vi "intake-shooter.vi"() -> ()   [LabVIEW 2023]
uses:
  ctrl defs/ctrl shooter speeds.ctl
  ctrl defs/ctrl intake speeds.ctl
  ctrl defs/ctrl INTAKE STATES.ctl
  ctrl defs/ctrl SHOOTER STATES.ctl
  <vilib>/Rock Robotics/WPI/MotorControl/WPI_MotorControlDeviceRef.ctl
  <vilib>/Rock Robotics/WPI/MotorControl/WPI_MotorControlType.ctl
  <vilib>/Rock Robotics/SystemInterfaces/DIO/FPGA_DIOPWMChannel.ctl
  <vilib>/Rock Robotics/WPI/PWM/WPI_PWMDeadband.ctl
  <vilib>/Rock Robotics/SystemInterfaces/DIO/FPGA_DIOChannel.ctl
  <vilib>/Rock Robotics/WPI/ThirdParty/REV Robotics/REVLib/Typedef/Spark MAX Control Type.ctl
  Global INIT.vi
  Global stack names.vi
  <vilib>/Rock Robotics/Network Tables/NT Write String.vi
  <vilib>/Rock Robotics/Network Tables/NT Read Boolean.vi
  <vilib>/Rock Robotics/Network Tables/NT Write Boolean.vi
panel:
  in  "AUTO run\nINTAKE after\nSHOT":bool
  in  "WRITE to global":bool
  in  "reload global values":bool
  in  "LOADER speeds":T1={"forward"=0.64, "reverse"=-1.0} {"reverse" min=-1.0 max=-0.02 format="%.3f"; "forward" min=0.02 max=1.0 format="%.3f"}
  in  "LOADER max/min":T1={"forward"=0.75, "reverse"=-0.75} {"reverse" min=-1.0 max=-0.02 format="%.3f"; "forward" min=0.02 max=1.0 format="%.3f"}
  in  "INTAKE speeds":T1={"forward"=1.0, "reverse"=-0.75} {"reverse" min=-1.0 max=-0.02 format="%.3f"; "forward" min=0.02 max=1.0 format="%.3f"}
  in  "SHOOTER speeds":T2={"SPEAKER"=1.0, "AMP"=0.5} {"AMP" min=0.02 max=1.0 format="%.3f"; "SPEAKER" min=0.02 max=1.0 format="%.3f"}
  in  "milliseconds to wait\nREV LOADER":u32=125
  in  "wait for SHOOT\nto end (ms)":u32=500
  in  "wait to\nSPIN UP\nSHOOTER (ms)":u32=250
  in  "OVERIDE\nNOTE check for\nSHOOT":bool
  out "LOOKING\nfor NOTE":bool
  out "note sensor":bool
  in  "SHOOT STATUS":string="STANDBY"
  out "% TARGET\nSPEED":dbl=-0.0
  out "Set SHOOTER\nRPM":dbl=1419.0 format="%#_13g"
  out "max rpm\n- SHOOTER":dbl=1419.0
  out "FIRE!":bool
  in  "INTAKE STATUS":string="Standby"
  out "max rpm\n- INTAKE":dbl=1419.0
  out "NOTE is\nloaded":bool
  out "run reverse":bool
  out "run intake":bool
  out "run? is\nACTIVE":bool
  in  "milliseconds to wait\nIN REVERSE":u32=1000
  in  "milliseconds to wait\nafter NOTE trigger":u32=25
  out "EXT FLAP":bool
  out "AMP OPT":bool
  in  "REVS to\nSHOOT":dbl=5.0 format="%#_13g"
  in  "REVS to\nRETRACT":dbl=-1.0 format="%#_13g"
  out "max rpm\n- LOADER":dbl=1419.0
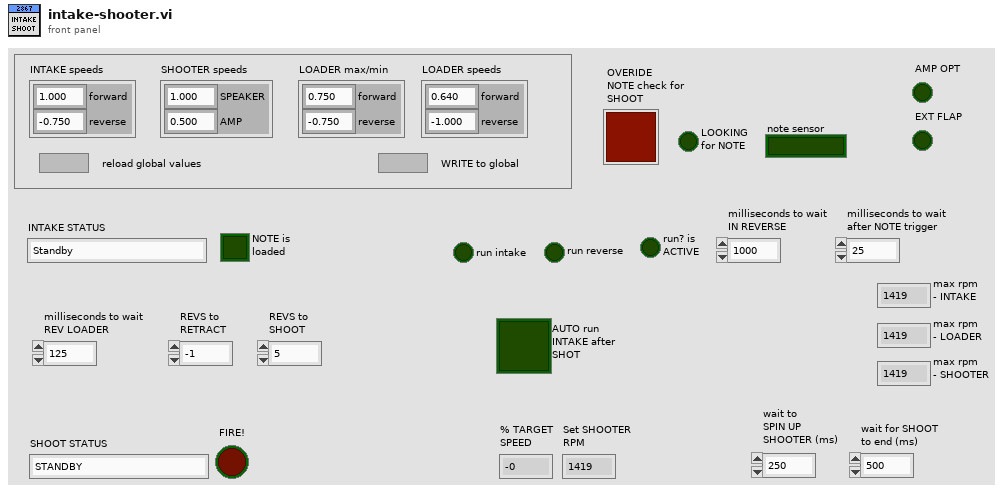
[diagram p1: front panel]
types:
  T1 = typedef "ctrl intake speeds.ctl" = cluster{"forward":dbl, "reverse":dbl}
  T2 = typedef "ctrl shooter speeds.ctl" = cluster{"SPEAKER":dbl, "AMP":dbl}
  T3 = typedef "ctrl SHOOTER STATES.ctl" = enum16{"STANDBY", "RETRACT NOTE", "SPIN-UP", "SHOOT", "RESET"}
  T4 = typedef "ctrl INTAKE STATES.ctl" = enum16{"STANDBY", "START INTAKES", "WATCH for NOTE", "SHUT DOWN", "REVERSE"}
  T5 = typedef "WPI_MotorControlDeviceRef.ctl" = cluster{"DeviceStatus":errorcluster, "Type":T6, "PWM":cluster{"PWM Channel":T7, "DeadBand":T8}, "CAN":cluster{"Device Number":u8, "SetOutput VI Ref":variant, "GetOutput VI Ref":variant, "Enable VI Ref":variant, "Disable VI Ref":variant, "Data":variant}, "Invert":bool, "DIO PWM":cluster{"PWM \"Enable\" Channel":T7, "DIOChannel":T9, "PWM Rate":dbl}}
  T6 = typedef "WPI_MotorControlType.ctl" = enum16{"PWM", "CAN", "DIO PWM"}
  T7 = typedef "FPGA_DIOPWMChannel.ctl" = enum8{"PWM 0", "PWM 1", "PWM 2", "PWM 3", "PWM 4", "PWM 5", "PWM 6", "PWM 7", "PWM 8", "PWM 9", "PWM MXP 0", "PWM MXP 1", "PWM MXP 2", "PWM MXP 3", "PWM MXP 4", "PWM MXP 5", "PWM MXP 6", "PWM MXP 7", "PWM MXP 8", "PWM MXP 9", "Invalid"}
  T8 = typedef "WPI_PWMDeadband.ctl" = cluster{"Name":string, "maxPositivePwm":i32, "minPositivePwm":i32, "centerPwm":i32, "maxNegativePwm":i32, "minNegativePwm":i32, "angularRange":u16}
  T9 = typedef "FPGA_DIOChannel.ctl" = enum8{"DIO 0", "DIO 1", "DIO 2", "DIO 3", "DIO 4", "DIO 5", "DIO 6", "DIO 7", "DIO 8", "DIO 9", "DIO MXP 0", "DIO MXP 1", "DIO MXP 2", "DIO MXP 3", "DIO MXP 4", "DIO MXP 5", "DIO MXP 6", "DIO MXP 7", "DIO MXP 8", "DIO MXP 9", "DIO MXP 10", "DIO MXP 11", "DIO MXP 12", "DIO MXP 13", "DIO MXP 14", "DIO MXP 15", "SPI Port CS1", "SPI Port CS2", "SPI Port CS3", "SPI Port MISO", "SPI Port MOSI", "Invalid"}
  T10 = cluster{"INTAKE ref":T5, "LOADER ref":T5, "SHOOTER ref":T5}
  T11 = typedef "ctrl DIO.ctl" = cluster{"description":string, "Installed?":bool, "DIOChannel":T9, "refnum name":string}
  T12 = typedef "ctrl swerve motor.ctl" = cluster{"description":string, "MOTOR SELECT":T13, "Installed?":bool, "CAN ID":u8, "refnum name":string, "Invert":bool, "Idle Mode":T14, "Current limiting":T15, "MOTOR PIDF coefficients":T16, "gear ratio":dbl}
  T13 = typedef "ctrl MOTOR SELECT.ctl" = i16
  T14 = typedef "Spark MAX Idle Mode.ctl" = enum16{"Coast", "Brake"}
  T15 = typedef "ctrl Spark MAX current limiting.ctl" = cluster{"Linearized":bool, "Free Speed (A)":dbl, "Primay (A)":dbl, "Limit RPM (0)":u32}
  T16 = typedef "ctrl motor PIDF coefficients.ctl" = cluster{"PIDF":cluster{"P Gain":dbl, "I Gain":dbl, "D Gain":dbl, "F Gain":dbl, "I Zone":dbl, "Min Output":dbl, "Max Output":dbl}, "Smart Motion":T17}
  T17 = typedef "Spark MAX Smart Motion Parameters.ctl" = cluster{"Max Velocity":dbl, "Max Acceleration":dbl, "Minimum Velocity Output":dbl, "Allowed Closed Loop Error":dbl}
  T18 = typedef "WPI_DigitalInputDevRef.ctl" = cluster{"DevStatus":errorcluster, "DIO Channel":T9}
  T19 = typedef "ctrl stack - INTAKE SHOOTER.ctl" = cluster{"INTAKE STATE":string, "RUN INTAKE?":string, "RUN REVERSE?":string, "NOTE LOADED?":string, "SHOOTER STATE":string, "SHOOTER FIRE?":string, "SHOOT AMP?":string, "EXTEND FLAP?":string, "LOOKING for NOTE":string}
  T20 = typedef "Spark MAX Control Type.ctl" = enum16{"Percent VBus", "Voltage", "Velocity", "Position", "Smart Motion", "Current", "Smart Velocity"}
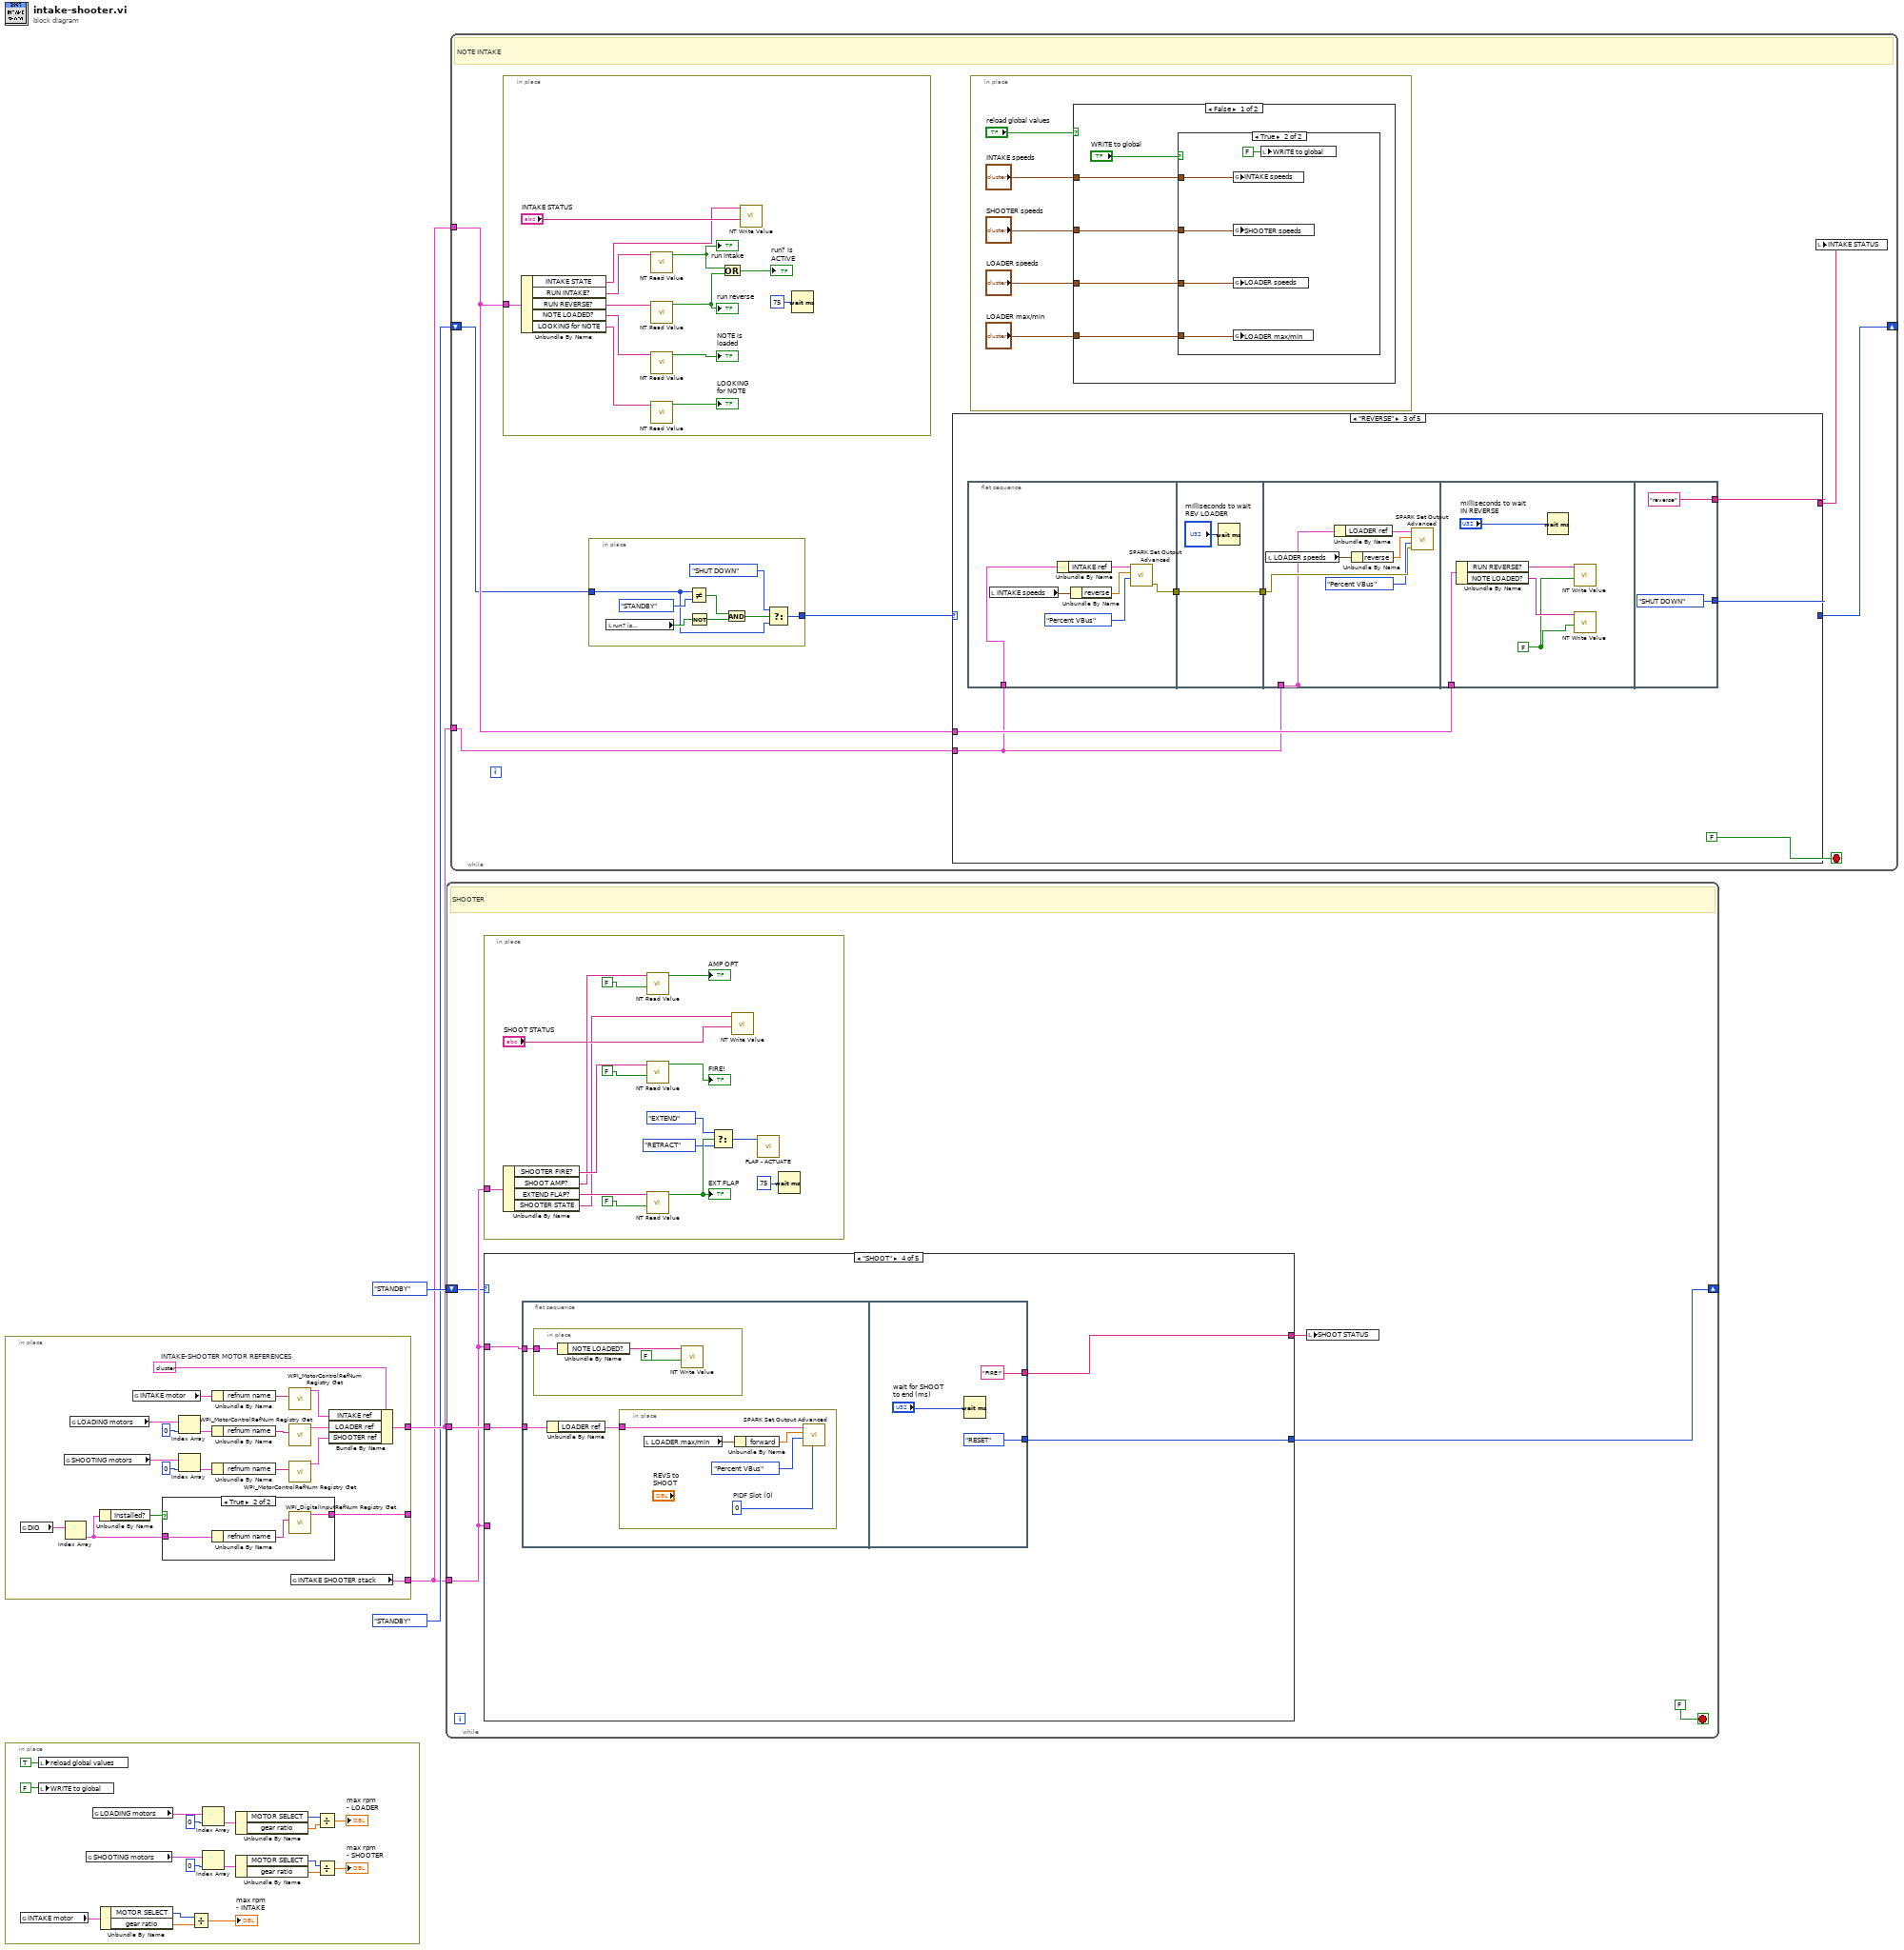
[diagram p0: block diagram]
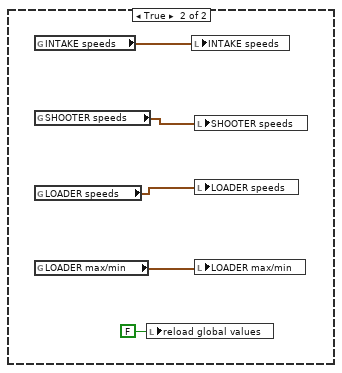
[diagram p3: hidden frame]
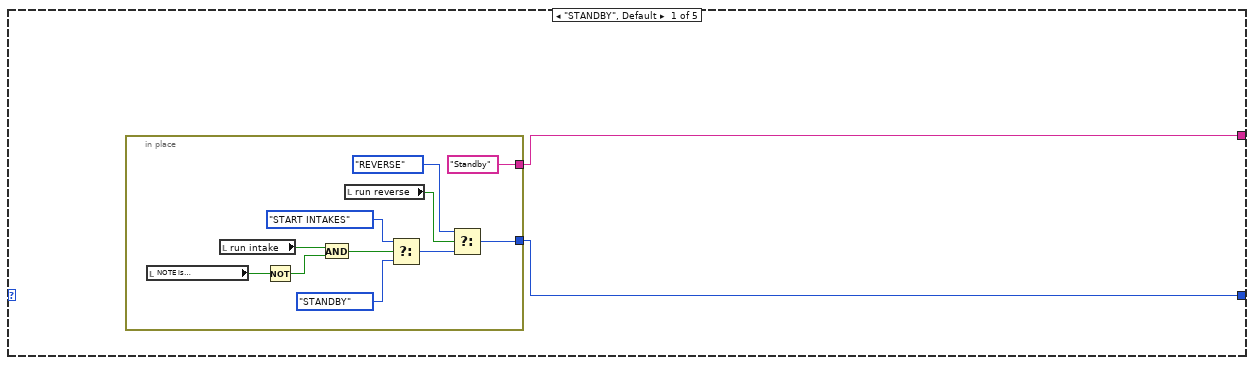
[diagram p4: hidden frame]
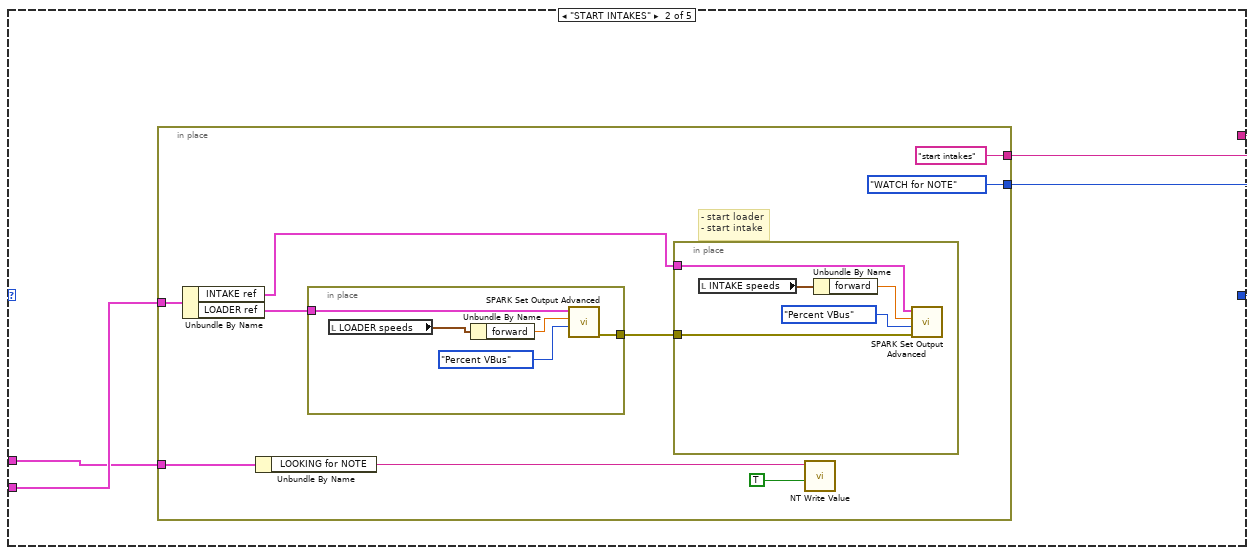
[diagram p5: hidden frame]
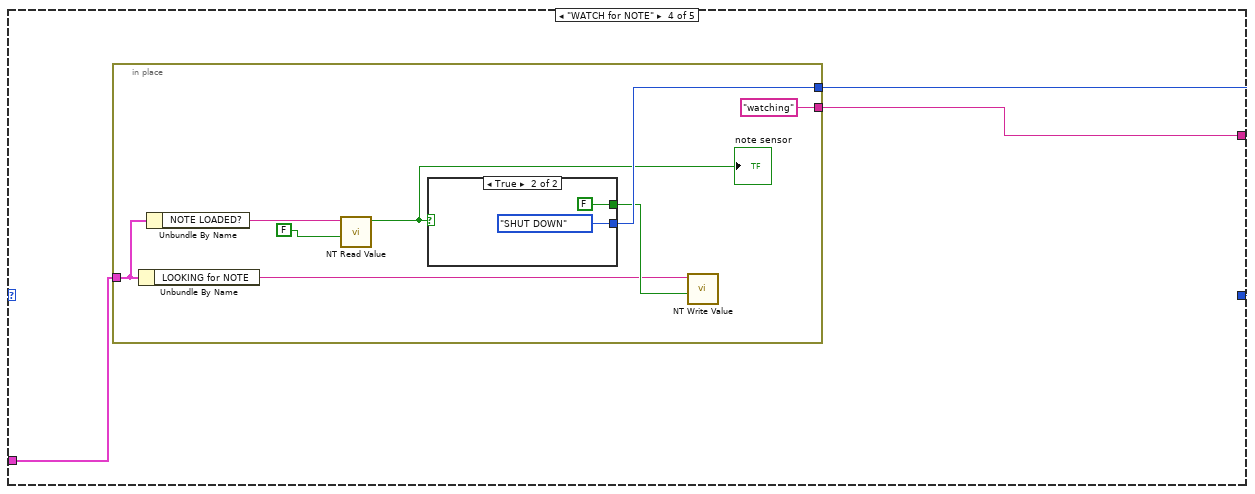
[diagram p6: hidden frame]
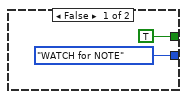
[diagram p7: hidden frame]
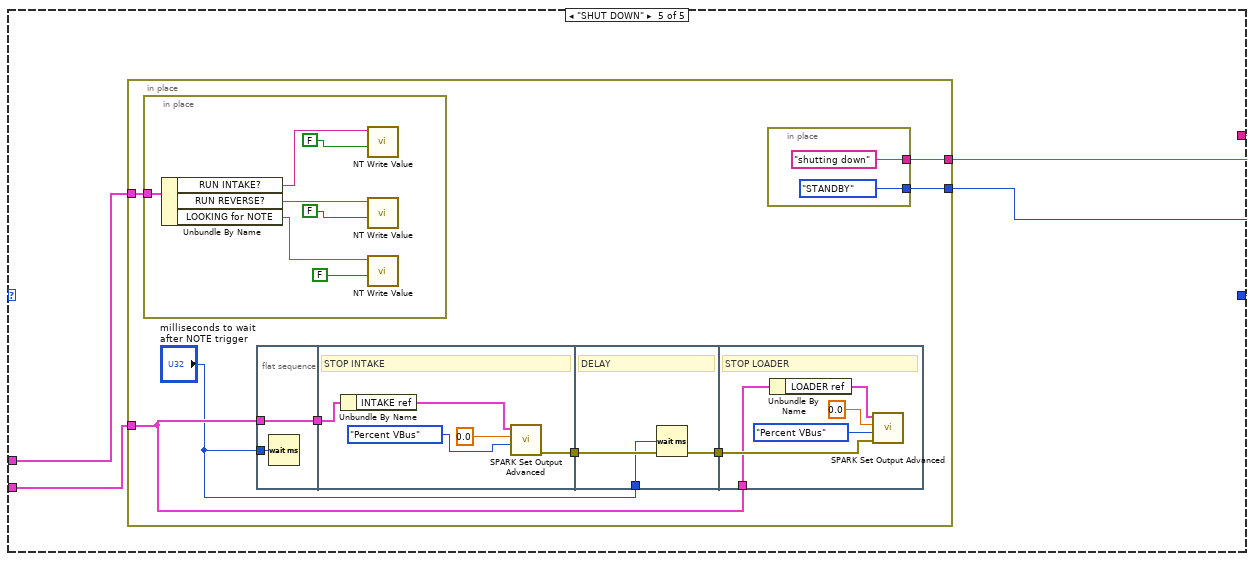
[diagram p8: hidden frame]
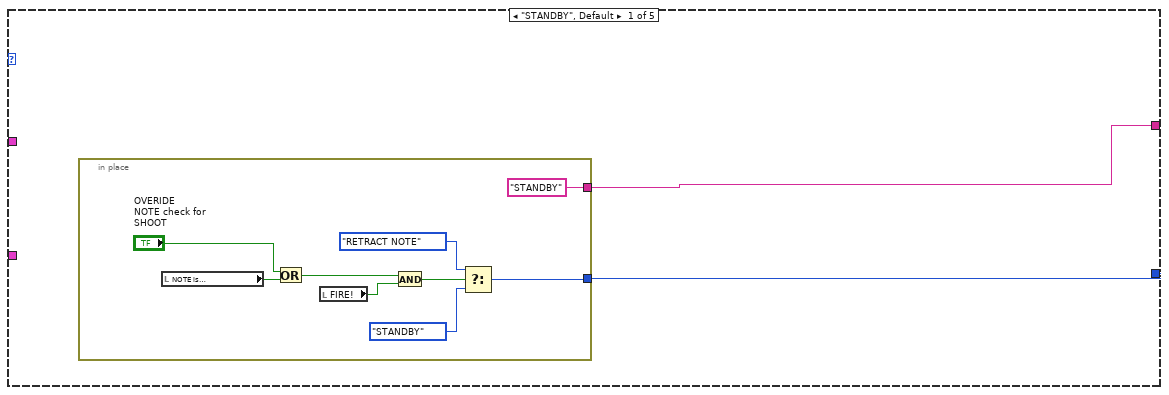
[diagram p9: hidden frame]
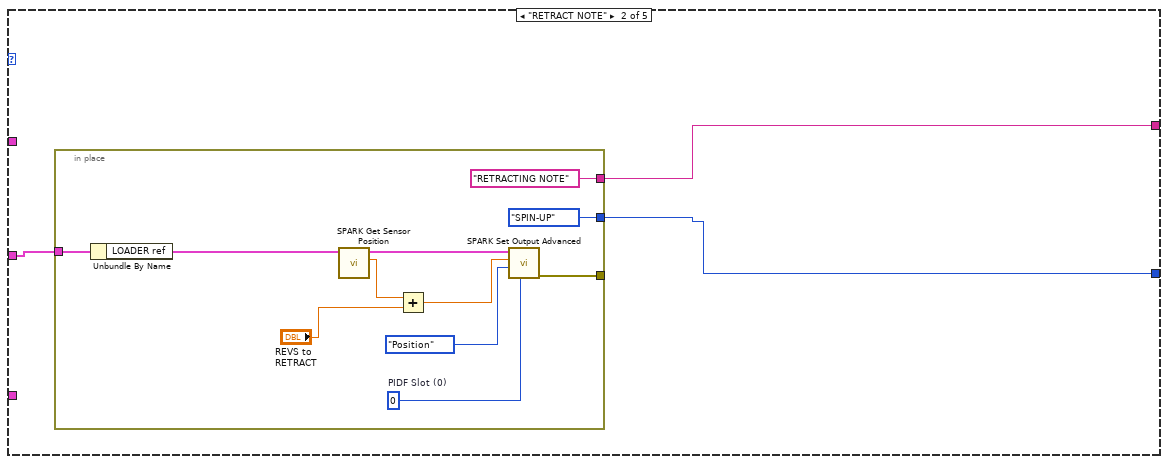
[diagram p10: hidden frame]
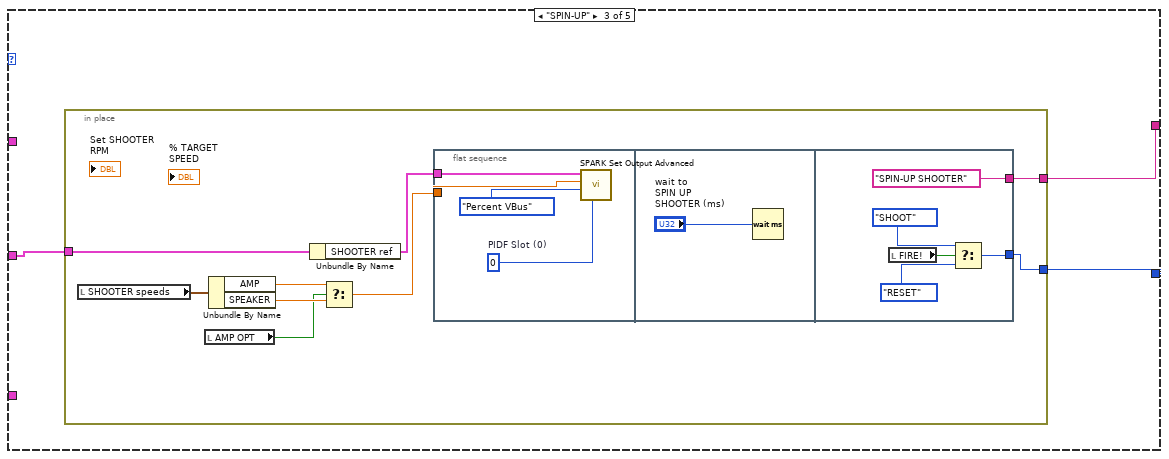
[diagram p11: hidden frame]
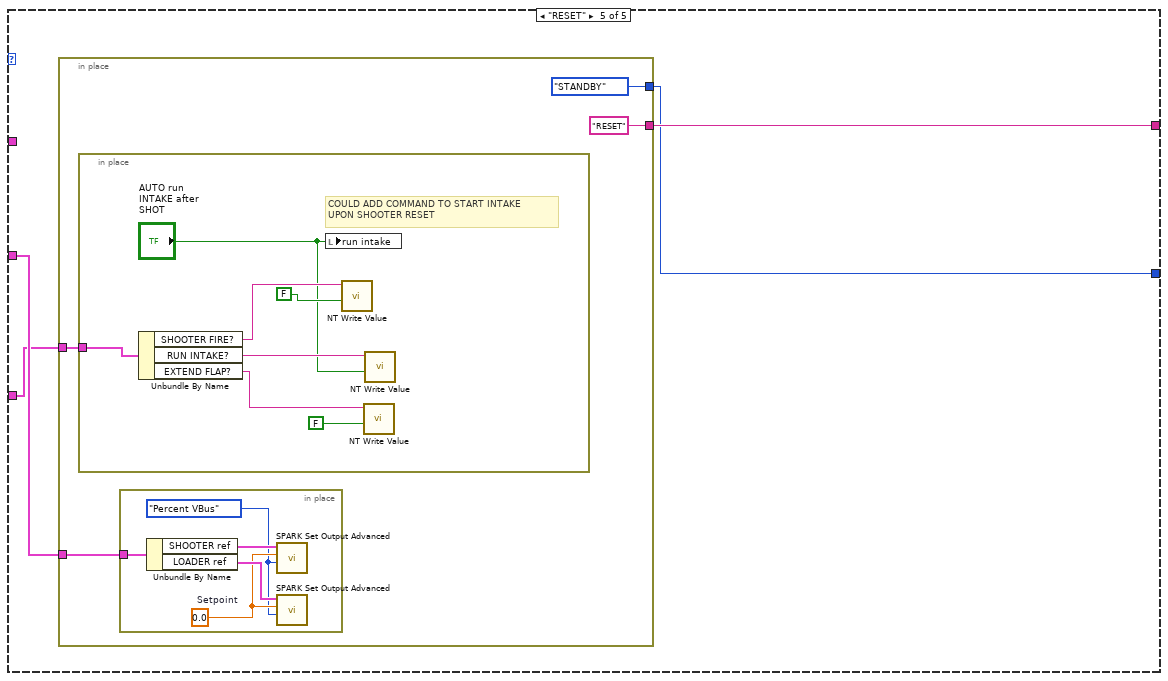
[diagram p12: hidden frame]
diagram:
  n1 = in-place {
    in-place-border: [w21] -> _
    in-place-border: [w6] -> w3
    in-place-border: [w5] -> w1
    w10 = T10 {"INTAKE ref"={"DeviceStatus"={"status"=FALSE, "code"=0, "source"=""}, "Type"=enum."PWM", "PWM"={"PWM Channel"=enum."Invalid", "DeadBand"={"Name"="", "maxPositivePwm"=0, "minPositivePwm"=0, "centerPwm"=0, "maxNegativePwm"=0, "minNegativePwm"=0, "angularRange"=0}}, "CAN"={"Device Number"=0, "SetOutput VI Ref"=variant(refnum<vi> refnum), "GetOutput VI Ref"=variant(refnum<vi> refnum), "Enable VI Ref"=variant(refnum<vi> refnum), "Disable VI Ref"=variant(refnum<vi> refnum), "Data"=variant}, "Invert"=FALSE, "DIO PWM"={"PWM \"Enable\" Channel"=enum."Invalid", "DIOChannel"=enum."Invalid", "PWM Rate"=0.0}}, "LOADER ref"={"DeviceStatus"={"status"=FALSE, "code"=0, "source"=""}, "Type"=enum."PWM", "PWM"={"PWM Channel"=enum."Invalid", "DeadBand"={"Name"="", "maxPositivePwm"=0, "minPositivePwm"=0, "centerPwm"=0, "maxNegativePwm"=0, "minNegativePwm"=0, "angularRange"=0}}, "CAN"={"Device Number"=0, "SetOutput VI Ref"=variant(refnum<vi> refnum), "GetOutput VI Ref"=variant(refnum<vi> refnum), "Enable VI Ref"=variant(refnum<vi> refnum), "Disable VI Ref"=variant(refnum<vi> refnum), "Data"=variant}, "Invert"=FALSE, "DIO PWM"={"PWM \"Enable\" Channel"=enum."Invalid", "DIOChannel"=enum."Invalid", "PWM Rate"=0.0}}, "SHOOTER ref"={"DeviceStatus"={"status"=FALSE, "code"=0, "source"=""}, "Type"=enum."PWM", "PWM"={"PWM Channel"=enum."Invalid", "DeadBand"={"Name"="", "maxPositivePwm"=0, "minPositivePwm"=0, "centerPwm"=0, "maxNegativePwm"=0, "minNegativePwm"=0, "angularRange"=0}}, "CAN"={"Device Number"=0, "SetOutput VI Ref"=variant(refnum<vi> refnum), "GetOutput VI Ref"=variant(refnum<vi> refnum), "Enable VI Ref"=variant(refnum<vi> refnum), "Disable VI Ref"=variant(refnum<vi> refnum), "Data"=variant}, "Invert"=FALSE, "DIO PWM"={"PWM \"Enable\" Channel"=enum."Invalid", "DIOChannel"=enum."Invalid", "PWM Rate"=0.0}}}  # INTAKE-SHOOTER MOTOR REFERENCES
    n2 = global read "Global INIT.vi" "DIO"() -> (w24:T11[])
    n3 = global read "Global INIT.vi" "SHOOTING motors"() -> (w19:T12[])
    n4 = Index Array(array=w24) -> (element=w22:T11)  [unwired: 1 in]
    n5 = global read "Global INIT.vi" "LOADING motors"() -> (w20:T12[])
    n6 = Unbundle By Name(w22) -> ("Installed?"=w23:bool)
    n7 = global read "Global INIT.vi" "INTAKE motor"() -> (w12:T12)
    n8 = case shown="True" w23 {
      tunnel: [_ w27] -> w21
      tunnel: w22 -> [_ w26]
      frame False {
      }
      frame True {
        n9 = Unbundle By Name(w26) -> ("refnum name"=w25:string)
        n10 = call <vilib>:"WPI_DigitalInputRefNum Registry Get.vi"("refnum name"=w25) -> ("DigitalInputDevRef"=w27:T18)  [unwired: 9 in, 1 out]
      }
    }
    n11 = Index Array(array=w20, index=0) -> (element=w16:T12)
    n12 = Index Array(array=w19, index=0) -> (element=w14:T12)
    n13 = Unbundle By Name(w12) -> ("refnum name"=w11:string)
    n14 = Unbundle By Name(w16) -> ("refnum name"=w15:string)
    n15 = Unbundle By Name(w14) -> ("refnum name"=w13:string)
    n16 = call <vilib>:"WPI_MotorControlRefNum Registry Get.vi"("refnum name"=w11) -> ("MotorControlDevRef"=w7:T5)  [unwired: 9 in, 1 out]
    n17 = call <vilib>:"WPI_MotorControlRefNum Registry Get.vi"("refnum name"=w15) -> ("MotorControlDevRef"=w8:T5)  [unwired: 9 in, 1 out]
    n18 = call <vilib>:"WPI_MotorControlRefNum Registry Get.vi"("refnum name"=w13) -> ("MotorControlDevRef"=w9:T5)  [unwired: 9 in, 1 out]
    n19 = global read "Global stack names.vi" "INTAKE SHOOTER stack"() -> (w5:T19)
    n20 = Bundle By Name(cluster=w10, "INTAKE ref"=w7, "LOADER ref"=w8, "SHOOTER ref"=w9) -> (w6:T10)
  }
  n21 = in-place {
    n22 = global read "Global INIT.vi" "INTAKE motor"() -> (w30:T12)
    n23 = local write "reload global values"(TRUE ("reload global values")) -> ()
    n24 = local write "WRITE to global"(FALSE ("WRITE to global")) -> ()
    n25 = global read "Global INIT.vi" "SHOOTING motors"() -> (w37:T12[])
    n26 = global read "Global INIT.vi" "LOADING motors"() -> (w42:T12[])
    n27 = Unbundle By Name(w30) -> ("MOTOR SELECT"=w32:T13, "gear ratio"=w31:dbl)
    n28 = Divide(x=w32, y=w31) -> (x/y=→"max rpm\n- INTAKE":dbl)
    n29 = Index Array(array=w42, index=0) -> (element=w40:T12)
    n30 = Index Array(array=w37, index=0) -> (element=w35:T12)
    n31 = Unbundle By Name(w40) -> ("MOTOR SELECT"=w39:T13, "gear ratio"=w38:dbl)
    n32 = Unbundle By Name(w35) -> ("MOTOR SELECT"=w34:T13, "gear ratio"=w33:dbl)
    n33 = Divide(x=w39, y=w38) -> (x/y=→"max rpm\n- LOADER":dbl)
    n34 = Divide(x=w34, y=w33) -> (x/y=→"max rpm\n- SHOOTER":dbl)
  }
  n35 = while {
    tunnel: w3 -> [w50]
    shift-right: [w51] -> _
    shift-left: ctrl_SHOOTER_STATES."STANDBY" -> [w46]
    tunnel: w1 -> [w47]
    stop <- FALSE stop-if-true
    # "SHOOTER"
    n36 = in-place {
      in-place-border: w47 -> [w151]
      n37 = Unbundle By Name(w151) -> ("SHOOTER FIRE?"=w150:string, "SHOOT AMP?"=w148:string, "EXTEND FLAP?"=w145:string, "SHOOTER STATE"=w138:string)
      n38 = call-poly <vilib>:"NT Read Value.vi"("default value"=FALSE, "name"=w148) -> ("value"=→"AMP OPT":bool)  [unwired: 7 in, 2 out]
      n39 = call-poly <vilib>:"NT Read Value.vi"("default value"=FALSE, "name"=w150) -> ("value"=→"FIRE!":bool)  [unwired: 7 in, 2 out]
      n40 = call-poly <vilib>:"NT Read Value.vi"("default value"=FALSE, "name"=w145) -> ("value"=w142:bool)  [unwired: 7 in, 2 out]
      "EXT FLAP" <- w142
      n41 = Select(t=enum16{"EXTEND", "RETRACT"}."EXTEND" ("STATE"), s=w142, f=enum16{"EXTEND", "RETRACT"}."RETRACT" ("STATE")) -> (s? t:f=w144:enum16{"EXTEND", "RETRACT"})
      n42 = call-poly <vilib>:"NT Write Value.vi"("value"="SHOOT STATUS", "name"=w138) -> ()  [unwired: 9 in, 1 out]
      n43 = call "FLAP - ACTUATE.vi"("STATE"=w144) -> ()  [unwired: 10 in, 1 out]
      n44 = Wait (ms)(milliseconds to wait=u32 75) -> ()  [unwired: 1 out]
    }
    n45 = case shown="\"SHOOT\"" w46 {
      tunnel: [w53 w64 w77 w99 w118] -> w51
      tunnel: w47 -> [_ _ _ w101 _]
      tunnel: w50 -> [_ w63 w79 w102 w120]
      tunnel: [w52 w65 w78 w100 w119] -> w49
      tunnel: w47 -> [_ _ _ _ w117]
      frame "STANDBY", Default {
        n46 = in-place {
          in-place-border: [w61] -> w53
          in-place-border: ["STANDBY" ("value")] -> w52
          n47 = local read "NOTE is\nloaded"() -> (w55:bool)
          n48 = Or(x="OVERIDE\nNOTE check for\nSHOOT", y=w55) -> (x .or. y?=w54:bool)
          n49 = local read "FIRE!"() -> (w59:bool)
          n50 = And(x=w54, y=w59) -> (x .and. y?=w60:bool)
          n51 = Select(t=ctrl_SHOOTER_STATES."RETRACT NOTE", s=w60, f=ctrl_SHOOTER_STATES."STANDBY") -> (s? t:f=w61:T3)
        }
      }
      frame "RETRACT NOTE" {
        n52 = in-place {
          in-place-border: ["RETRACTING NOTE" ("value")] -> w65
          in-place-border: [ctrl_SHOOTER_STATES."SPIN-UP"] -> w64
          in-place-border: [w69] -> _
          in-place-border: w63 -> [w68]
          w73 = 0  # PIDF Slot (0)
          n53 = Unbundle By Name(w68) -> ("LOADER ref"=w67:T5)
          n54 = call <vilib>:"SPARK Get Sensor Position.vi"("MotorControlDevRef in"=w67) -> ("Sensor Position"=w70:dbl, "MotorControlDevRef out"=w72:T5)  [unwired: 7 in, 2 out]
          n55 = Add(x=w70, y="REVS to\nRETRACT") -> (x+y=w71:dbl)
          n56 = call <vilib>:"SPARK Set Output Advanced.vi"("PIDF Slot (0)"=w73, "Control Mode"=Spark_MAX_Control_Type."Position", "Setpoint"=w71, "MotorControlDevRef"=w72) -> ("error out"=w69:errorcluster)  [unwired: 6 in, 1 out]
        }
      }
      frame "SPIN-UP" {
        n57 = in-place {
          in-place-border: w79 -> [w88]
          in-place-border: [w80] -> w78
          in-place-border: [w81] -> w77
          n58 = local read "SHOOTER speeds"() -> (w83:T2)
          n59 = local read "AMP OPT"() -> (w84:bool)
          n60 = Unbundle By Name(w83) -> ("AMP"=w85:dbl, "SPEAKER"=w86:dbl)
          n61 = Unbundle By Name(w88) -> ("SHOOTER ref"=w87:T5)
          n62 = Select(t=w85, s=w84, f=w86) -> (s? t:f=w82:dbl)
          n63 = flat-sequence {
            tunnel: w87 -> [w92]
            tunnel: w82 -> [w91]
            tunnel: [w96] -> w81
            tunnel: ["SPIN-UP SHOOTER" ("value")] -> w80
            frame #0 {
              w89 = 0  # PIDF Slot (0)
              n64 = call <vilib>:"SPARK Set Output Advanced.vi"("PIDF Slot (0)"=w89, "Control Mode"=Spark_MAX_Control_Type."Percent VBus", "Setpoint"=w91, "MotorControlDevRef"=w92) -> ()  [unwired: 6 in, 2 out]
            }
            frame #1 {
              n65 = Wait (ms)(milliseconds to wait="wait to\nSPIN UP\nSHOOTER (ms)") -> ()  [unwired: 1 out]
            }
            frame #2 {
              n66 = local read "FIRE!"() -> (w98:bool)
              n67 = Select(t=ctrl_SHOOTER_STATES."SHOOT", s=w98, f=ctrl_SHOOTER_STATES."RESET") -> (s? t:f=w96:T3)
            }
          }
        }
      }
      frame "SHOOT" {
        n68 = flat-sequence {
          tunnel: w102 -> [w105]
          tunnel: w101 -> [w103]
          tunnel: [ctrl_SHOOTER_STATES."RESET"] -> w99
          tunnel: ["FIRE!" ("value")] -> w100
          frame #0 {
            n69 = in-place {
              in-place-border: w103 -> [w113]
              n70 = Unbundle By Name(w113) -> ("NOTE LOADED?"=w112:string)
              n71 = call-poly <vilib>:"NT Write Value.vi"("value"=FALSE, "name"=w112) -> ()  [unwired: 9 in, 1 out]
            }
            n72 = Unbundle By Name(w105) -> ("LOADER ref"=w104:T5)
            n73 = in-place {
              in-place-border: w104 -> [w110]
              w109 = 0  # PIDF Slot (0)
              n74 = local read "LOADER max/min"() -> (w107:T1)
              n75 = Unbundle By Name(w107) -> ("forward"=w106:dbl)
              n76 = call <vilib>:"SPARK Set Output Advanced.vi"("PIDF Slot (0)"=w109, "Control Mode"=Spark_MAX_Control_Type."Percent VBus", "Setpoint"=w106, "MotorControlDevRef"=w110) -> ()  [unwired: 6 in, 2 out]
            }
          }
          frame #1 {
            n77 = Wait (ms)(milliseconds to wait="wait for SHOOT\nto end (ms)") -> ()  [unwired: 1 out]
          }
        }
      }
      frame "RESET" {
        n78 = in-place {
          in-place-border: w120 -> [w124]
          in-place-border: ["RESET" ("value")] -> w119
          in-place-border: [ctrl_SHOOTER_STATES."STANDBY"] -> w118
          in-place-border: w117 -> [w121]
          n79 = in-place {
            in-place-border: w121 -> [w135]
            # "COULD ADD COMMAND TO START INTAKE\nUPON SHOOTER RESET"
            n80 = Unbundle By Name(w135) -> ("SHOOTER FIRE?"=w134:string, "RUN INTAKE?"=w133:string, "EXTEND FLAP?"=w131:string)
            n81 = local write "run intake"("AUTO run\nINTAKE after\nSHOT") -> ()
            n82 = call-poly <vilib>:"NT Write Value.vi"("value"=FALSE ("default value"), "name"=w134) -> ()  [unwired: 9 in, 1 out]
            n83 = call-poly <vilib>:"NT Write Value.vi"("value"=FALSE, "name"=w131) -> ()  [unwired: 9 in, 1 out]
            n84 = call-poly <vilib>:"NT Write Value.vi"("value"="AUTO run\nINTAKE after\nSHOT", "name"=w133) -> ()  [unwired: 9 in, 1 out]
          }
          n85 = in-place {
            in-place-border: w124 -> [w127]
            w126 = 0.0  # Setpoint
            w125 = Spark_MAX_Control_Type."Percent VBus" ("Control Mode")
            n86 = Unbundle By Name(w127) -> ("SHOOTER ref"=w128:T5, "LOADER ref"=w129:T5)
            n87 = call <vilib>:"SPARK Set Output Advanced.vi"("Control Mode"=w125, "Setpoint"=w126, "MotorControlDevRef"=w128) -> ()  [unwired: 7 in, 2 out]
            n88 = call <vilib>:"SPARK Set Output Advanced.vi"("Control Mode"=w125, "Setpoint"=w126, "MotorControlDevRef"=w129) -> ()  [unwired: 7 in, 2 out]
          }
        }
      }
    }
    n89 = local write "SHOOT STATUS"(w49) -> ()
  }
  n90 = while {
    shift-right: [w158] -> _
    shift-left: ctrl_INTAKE_STATES."STANDBY" ("INTAKE STATE") -> [w155]
    tunnel: w3 -> [w157]
    tunnel: w1 -> [w156]
    stop <- FALSE stop-if-true
    # "NOTE INTAKE"
    n91 = in-place {
      in-place-border: w156 -> [w309]
      n92 = Unbundle By Name(w309) -> ("INTAKE STATE"=w304:string, "RUN INTAKE?"=w311:string, "RUN REVERSE?"=w310:string, "NOTE LOADED?"=w312:string, "LOOKING for NOTE"=w301:string)
      n93 = call-poly <vilib>:"NT Read Value.vi"("name"=w311) -> ("value"=w308:bool)  [unwired: 8 in, 2 out]
      "run intake" <- w308
      n94 = call-poly <vilib>:"NT Read Value.vi"("name"=w310) -> ("value"=w307:bool)  [unwired: 8 in, 2 out]
      "run reverse" <- w307
      n95 = call-poly <vilib>:"NT Read Value.vi"("name"=w312) -> ("value"=→"NOTE is\nloaded":bool)  [unwired: 8 in, 2 out]
      n96 = call-poly <vilib>:"NT Read Value.vi"("name"=w301) -> ("value"=→"LOOKING\nfor NOTE":bool)  [unwired: 8 in, 2 out]
      n97 = Or(x=w308, y=w307) -> (x .or. y?=→"run? is\nACTIVE":bool)
      n98 = call-poly <vilib>:"NT Write Value.vi"("value"="INTAKE STATUS", "name"=w304) -> ()  [unwired: 9 in, 1 out]
      n99 = Wait (ms)(milliseconds to wait=u32 75) -> ()  [unwired: 1 out]
    }
    n100 = in-place {
      in-place-border: w155 -> [w180]
      in-place-border: [w183] -> w154
      n101 = local read "run? is\nACTIVE"() -> (w184:bool)
      n102 = Not Equal?(x=w180, y=ctrl_INTAKE_STATES."STANDBY" ("INTAKE STATE")) -> (x != y?=w187:bool)
      n103 = Not(x=w184) -> (.not. x?=w185:bool)
      n104 = And(x=w187, y=w185) -> (x .and. y?=w181:bool)
      n105 = Select(t=ctrl_INTAKE_STATES."SHUT DOWN" ("INTAKE STATE"), s=w181, f=w180) -> (s? t:f=w183:T4)
    }
    n106 = case shown="\"REVERSE\"" w154 {
      tunnel: [w189 w204 w228 w252 w269] -> w158
      tunnel: [w188 w203 w227 w253 w268] -> w153
      tunnel: w157 -> [_ w202 w224 _ w267]
      tunnel: w156 -> [_ w201 w229 w251 w266]
      frame "STANDBY", Default {
        n107 = in-place {
          in-place-border: [w195] -> w189
          in-place-border: ["Standby" ("value")] -> w188
          n108 = local read "NOTE is\nloaded"() -> (w192:bool)
          n109 = local read "run intake"() -> (w191:bool)
          n110 = Not(x=w192) -> (.not. x?=w198:bool)
          n111 = And(x=w191, y=w198) -> (x .and. y?=w199:bool)
          n112 = local read "run reverse"() -> (w193:bool)
          n113 = Select(t=ctrl_INTAKE_STATES."START INTAKES" ("INTAKE STATE 2"), s=w199, f=ctrl_INTAKE_STATES."STANDBY" ("INTAKE STATE 2")) -> (s? t:f=w196:T4)
          n114 = Select(t=ctrl_INTAKE_STATES."REVERSE" ("INTAKE STATE 2"), s=w193, f=w196) -> (s? t:f=w195:T4)
        }
      }
      frame "START INTAKES" {
        n115 = in-place {
          in-place-border: [ctrl_INTAKE_STATES."WATCH for NOTE" ("INTAKE STATE 2")] -> w204
          in-place-border: ["start intakes" ("value")] -> w203
          in-place-border: w202 -> [w211]
          in-place-border: w201 -> [w206]
          # "- start loader\n- start intake"
          n116 = Unbundle By Name(w211) -> ("INTAKE ref"=w210:T5, "LOADER ref"=w209:T5)
          n117 = Unbundle By Name(w206) -> ("LOOKING for NOTE"=w207:string)
          n118 = in-place {
            in-place-border: w209 -> [w218]
            in-place-border: [w216] -> w208
            n119 = local read "LOADER speeds"() -> (w214:T1)
            n120 = Unbundle By Name(w214) -> ("forward"=w215:dbl)
            n121 = call <vilib>:"SPARK Set Output Advanced.vi"("Control Mode"=Spark_MAX_Control_Type."Percent VBus", "Setpoint"=w215, "MotorControlDevRef"=w218) -> ("error out"=w216:errorcluster)  [unwired: 7 in, 1 out]
          }
          n122 = in-place {
            in-place-border: w210 -> [w223]
            in-place-border: w208 -> [w221]
            n123 = local read "INTAKE speeds"() -> (w220:T1)
            n124 = Unbundle By Name(w220) -> ("forward"=w219:dbl)
            n125 = call <vilib>:"SPARK Set Output Advanced.vi"("error in (no error)"=w221, "Control Mode"=Spark_MAX_Control_Type."Percent VBus", "Setpoint"=w219, "MotorControlDevRef"=w223) -> ()  [unwired: 6 in, 2 out]
          }
          n126 = call-poly <vilib>:"NT Write Value.vi"("value"=TRUE, "name"=w207) -> ()  [unwired: 9 in, 1 out]
        }
      }
      frame "REVERSE" {
        n127 = flat-sequence {
          tunnel: w224 -> [w233]
          tunnel: [w230] -> w226
          tunnel: w226 -> [w237]
          tunnel: [w237] -> w225
          tunnel: w225 -> [w243]
          tunnel: [w239] -> _
          tunnel: w224 -> [w239]
          tunnel: w229 -> [w247]
          tunnel: [ctrl_INTAKE_STATES."SHUT DOWN" ("INTAKE STATE 2")] -> w228
          tunnel: ["reverse" ("value")] -> w227
          frame #0 {
            n128 = local read "INTAKE speeds"() -> (w232:T1)
            n129 = Unbundle By Name(w233) -> ("INTAKE ref"=w235:T5)
            n130 = Unbundle By Name(w232) -> ("reverse"=w231:dbl)
            n131 = call <vilib>:"SPARK Set Output Advanced.vi"("Control Mode"=Spark_MAX_Control_Type."Percent VBus", "Setpoint"=w231, "MotorControlDevRef"=w235) -> ("error out"=w230:errorcluster)  [unwired: 7 in, 1 out]
          }
          frame #1 {
            n132 = Wait (ms)(milliseconds to wait="milliseconds to wait\nREV LOADER") -> ()  [unwired: 1 out]
          }
          frame #2 {
            n133 = local read "LOADER speeds"() -> (w242:T1)
            n134 = Unbundle By Name(w239) -> ("LOADER ref"=w238:T5)
            n135 = Unbundle By Name(w242) -> ("reverse"=w241:dbl)
            n136 = call <vilib>:"SPARK Set Output Advanced.vi"("error in (no error)"=w243, "Control Mode"=Spark_MAX_Control_Type."Percent VBus", "Setpoint"=w241, "MotorControlDevRef"=w238) -> ()  [unwired: 6 in, 2 out]
          }
          frame #3 {
            w245 = FALSE ("value")
            n137 = Unbundle By Name(w247) -> ("RUN REVERSE?"=w244:string, "NOTE LOADED?"=w248:string)
            n138 = Wait (ms)(milliseconds to wait="milliseconds to wait\nIN REVERSE") -> ()  [unwired: 1 out]
            n139 = call-poly <vilib>:"NT Write Value.vi"("value"=w245, "name"=w244) -> ()  [unwired: 9 in, 1 out]
            n140 = call-poly <vilib>:"NT Write Value.vi"("value"=w245, "name"=w248) -> ()  [unwired: 9 in, 1 out]
          }
          frame #4 {
          }
        }
      }
      frame "WATCH for NOTE" {
        n141 = in-place {
          in-place-border: ["watching" ("value")] -> w253
          in-place-border: [w260] -> w252
          in-place-border: w251 -> [w257]
          n142 = Unbundle By Name(w257) -> ("LOOKING for NOTE"=w254:string)
          n143 = Unbundle By Name(w257) -> ("NOTE LOADED?"=w258:string)
          n144 = call-poly <vilib>:"NT Read Value.vi"("default value"=FALSE ("value"), "name"=w258) -> ("value"=w256:bool)  [unwired: 7 in, 2 out]
          "note sensor" <- w256
          n145 = case shown="True" w256 {
            tunnel: [ctrl_INTAKE_STATES."WATCH for NOTE" ("INTAKE STATE 2") ctrl_INTAKE_STATES."SHUT DOWN" ("INTAKE STATE 2")] -> w260
            tunnel: [TRUE ("value") FALSE ("value")] -> w255
            frame False {
            }
            frame True {
            }
          }
          n146 = call-poly <vilib>:"NT Write Value.vi"("value"=w255, "name"=w254) -> ()  [unwired: 9 in, 1 out]
        }
      }
      frame "SHUT DOWN" {
        n147 = in-place {
          in-place-border: [w275] -> w269
          in-place-border: [w274] -> w268
          in-place-border: w267 -> [w273]
          in-place-border: w266 -> [w272]
          n148 = in-place {
            in-place-border: w272 -> [w298]
            n149 = Unbundle By Name(w298) -> ("RUN INTAKE?"=w297:string, "RUN REVERSE?"=w296:string, "LOOKING for NOTE"=w295:string)
            n150 = call-poly <vilib>:"NT Write Value.vi"("value"=FALSE, "name"=w297) -> ()  [unwired: 9 in, 1 out]
            n151 = call-poly <vilib>:"NT Write Value.vi"("value"=FALSE, "name"=w296) -> ()  [unwired: 9 in, 1 out]
            n152 = call-poly <vilib>:"NT Write Value.vi"("value"=FALSE, "name"=w295) -> ()  [unwired: 9 in, 1 out]
          }
          n153 = flat-sequence {
            tunnel: w273 -> [w279]
            tunnel: [w279] -> w271
            tunnel: "milliseconds to wait\nafter NOTE trigger" -> [w278]
            tunnel: [w284] -> w277
            tunnel: w271 -> [w283]
            tunnel: w277 -> [w286]
            tunnel: [w286] -> w276
            tunnel: "milliseconds to wait\nafter NOTE trigger" -> [w285]
            tunnel: w276 -> [w290]
            tunnel: w273 -> [w287]
            frame #0 {
              n154 = Wait (ms)(milliseconds to wait=w278) -> ()  [unwired: 1 out]
            }
            frame #1 {
              # "STOP INTAKE"
              n155 = Unbundle By Name(w283) -> ("INTAKE ref"=w280:T5)
              n156 = call <vilib>:"SPARK Set Output Advanced.vi"("Control Mode"=Spark_MAX_Control_Type."Percent VBus", "Setpoint"=0.0, "MotorControlDevRef"=w280) -> ("error out"=w284:errorcluster)  [unwired: 7 in, 1 out]
            }
            frame #2 {
              # "DELAY"
              n157 = Wait (ms)(milliseconds to wait=w285) -> ()  [unwired: 1 out]
            }
            frame #3 {
              # "STOP LOADER"
              n158 = Unbundle By Name(w287) -> ("LOADER ref"=w291:T5)
              n159 = call <vilib>:"SPARK Set Output Advanced.vi"("error in (no error)"=w290, "Control Mode"=Spark_MAX_Control_Type."Percent VBus", "Setpoint"=0.0, "MotorControlDevRef"=w291) -> ()  [unwired: 6 in, 2 out]
            }
          }
          n160 = in-place {
            in-place-border: [ctrl_INTAKE_STATES."STANDBY" ("INTAKE STATE 2")] -> w275
            in-place-border: ["shutting down" ("value")] -> w274
          }
        }
      }
    }
    n161 = in-place {
      n162 = case shown="False" "reload global values" {
        tunnel: "LOADER max/min" -> [w168 _]
        tunnel: "LOADER speeds" -> [w167 _]
        tunnel: "SHOOTER speeds" -> [w166 _]
        tunnel: "INTAKE speeds" -> [w165 _]
        frame False {
          n163 = case shown="True" "WRITE to global" {
            tunnel: w168 -> [_ w173]
            tunnel: w167 -> [_ w172]
            tunnel: w166 -> [_ w171]
            tunnel: w165 -> [_ w170]
            frame False {
            }
            frame True {
              n164 = global write "Global INIT.vi" "INTAKE speeds"(w170) -> ()
              n165 = global write "Global INIT.vi" "SHOOTER speeds"(w171) -> ()
              n166 = global write "Global INIT.vi" "LOADER speeds"(w172) -> ()
              n167 = global write "Global INIT.vi" "LOADER max/min"(w173) -> ()
              n168 = local write "WRITE to global"(FALSE ("WRITE to global")) -> ()
            }
          }
        }
        frame True {
          n169 = global read "Global INIT.vi" "INTAKE speeds"() -> (w178:T1)
          n170 = global read "Global INIT.vi" "SHOOTER speeds"() -> (w177:T2)
          n171 = global read "Global INIT.vi" "LOADER speeds"() -> (w176:T1)
          n172 = global read "Global INIT.vi" "LOADER max/min"() -> (w175:T1)
          n173 = local write "reload global values"(FALSE ("reload global values")) -> ()
          n174 = local write "INTAKE speeds"(w178) -> ()
          n175 = local write "SHOOTER speeds"(w177) -> ()
          n176 = local write "LOADER speeds"(w176) -> ()
          n177 = local write "LOADER max/min"(w175) -> ()
        }
      }
    }
    n178 = local write "INTAKE STATUS"(w153) -> ()
  }
